vi "util_queue_status.vi"(8 "error in (no error)":errorcluster) -> (0 "error out":errorcluster)   [LabVIEW 2015, in "lv-recipe-machine.lvlib"]
uses:
  lv-recipe-machine.lvlib
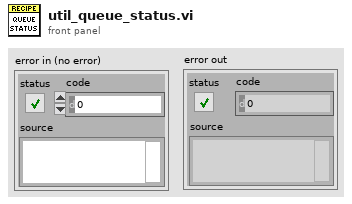
[diagram p1: front panel]
types:
  T1 = typedef "lv-recipe-machine.lvlib/references.ctl" = cluster{"semaphore":T2, "input_queue":refnum<queue>, "output_queue":refnum<queue>, "transition_queue":refnum<queue>, "data_dvr":refnum<data-value>, "stop_notifier":refnum<notifier>, "change_in_event":refnum<user-event>, "change_out_event":refnum<user-event>, "status_event":refnum<user-event>}
  T2 = typedef "Semaphore RefNum" = refnum<k1>
  T3 = typedef "lv-recipe-machine.lvlib/status.ctl" = cluster{"mode":T4, "manual_state":T5, "automatic_state":T6, "automatic_data":variant, "step":string, "recipe_elapsed_time":dbl, "step_elapsed_time":dbl, "recipe_error":errorcluster}
  T4 = typedef "lv-recipe-machine.lvlib/mode.ctl" = enum16{"<mode>", "manual", "automatic", "<null>"}
  T5 = typedef "lv-recipe-machine.lvlib/manual_state.ctl" = enum16{"<manual_state>", "failed", "action", "running", "idle", "<null>"}
  T6 = typedef "lv-recipe-machine.lvlib/automatic_state.ctl" = enum16{"<automatic_state>", "failed", "idle", "running", "paused", "stopped", "<null>"}
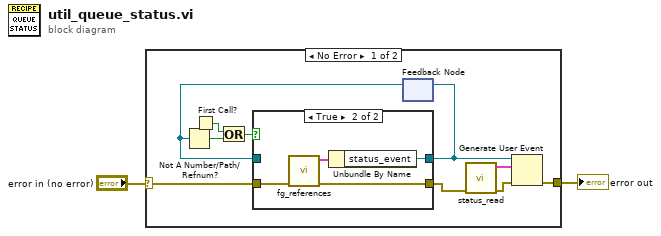
[diagram p0: block diagram]
diagram:
  n1 = case shown="No Error" "error in (no error)" {
    selector: "error in (no error)" -> [w5 w19]
    tunnel: [w12 w19] -> w2
    frame No Error {
      n2 = First Call?() -> (First Call?: T/F=w8:bool)
      n3 = feedback #1() -> (w7:refnum<user-event>)  [unwired: 1 in]
      n4 = Not A Number/Path/Refnum?(number/path/refnum=w7) -> (NaN/Path/Refnum?=w9:bool)
      n5 = Or(x=w8, y=w9) -> (x .or. y?=w6:bool)
      n6 = case shown="True" w6 {
        tunnel: w5 -> [w13 w18]
        tunnel: [w13 w17] -> w3
        tunnel: [w14 w15] -> w4
        tunnel: w7 -> [w14 _]
        frame False {
        }
        frame True {
          n7 = call "fg_references.vi"("error in (no error)"=w18) -> ("error out"=w17:errorcluster, "references out"=w16:T1)  [unwired: 9 in]
          n8 = Unbundle By Name(w16) -> ("status_event"=w15:refnum<user-event>)
        }
      }
      n9 = feedback-in #1(w4) -> ()
      n10 = call "status_read.vi"("error in (no error)"=w3) -> ("error out"=w10:errorcluster, "status"=w11:T3)  [unwired: 9 in]
      n11 = Generate User Event(user event=w4, event data cluster=w11, error in=w10) -> (error out=w12:errorcluster)  [unwired: 1 in, 1 out]
    }
    frame Error {
    }
  }
  "error out" <- w2
